vi "Laboratory_practice8.vi"() -> ()   [LabVIEW 2022 SP3]
uses:
  <vilib>/Analysis/3filter.llb/Butterworth Filter (DBL).vi
  <vilib>/Analysis/NI_AALBase.lvlib
panel:
  out "Peak to Peak":dbl
  in  "stop":bool
  out "RMS":dbl
  out "Waveform Graph":dynamicdata(graph)
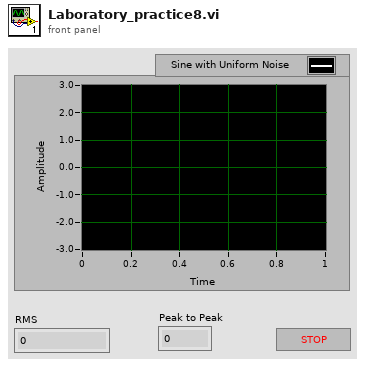
[diagram p1: front panel]
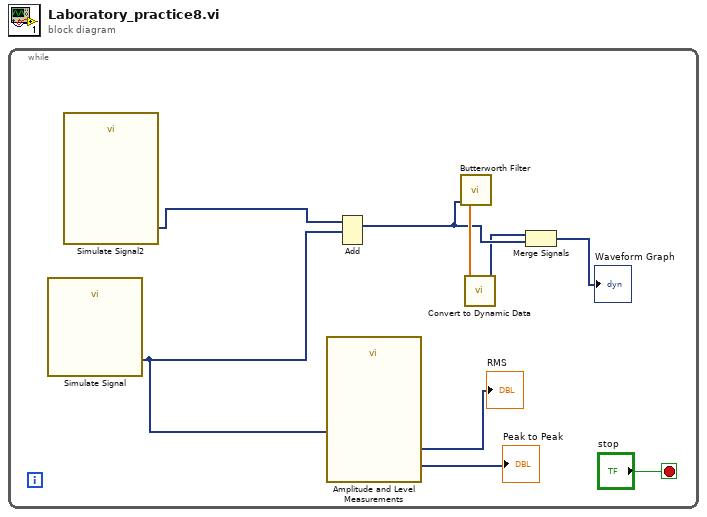
[diagram p0: block diagram]
diagram:
  n1 = while {
    stop <- "stop" stop-if-true
    n2 = call "Simulate Signal"() -> ("Sine"=w6:dynamicdata)  [unwired: 14 in, 1 out]
    n3 = call "Simulate Signal2"() -> ("Sine with Uniform Noise"=w5:dynamicdata)  [unwired: 14 in, 1 out]
    n4 = call "Amplitude and Level Measurements"("Signals"=w6) -> ("RMS"=→"RMS":dynamicdata, "Peak to Peak"=→"Peak to Peak":dynamicdata)  [unwired: 12 in, 1 out]
    n5 = Add(1:w6, 2:w5) -> (0:w2:dynamicdata)  [unwired: 1 in, 1 out]
    n6 = call-poly <vilib>:"Butterworth Filter.vi"("low cutoff freq: fl"=w2) -> ("Filtered X"=w4:dbl[])  [unwired: 7 in, 1 out]
    n7 = call "Convert to Dynamic Data"("Array"=w4) -> ("Dynamic Data Type"=w1:dynamicdata)  [unwired: 3 in]
    n8 = Merge Signals(w1, w2) -> (→"Waveform Graph":dynamicdata)
  }
